vi "Configure View Model.vi"(8 "error in (no error)":errorcluster, 10 "View Model":refnum<class "Multicolumn List Box View Model.lvclass">, 11 "Multicolumn List Box View In":refnum<class "Multicolumn List Box View.lvclass">) -> (0 "error out":errorcluster, 3 "Multicolumn List Box View Out":refnum<class "Multicolumn List Box View.lvclass">)   [LabVIEW 2020, in "Multicolumn List Box View.lvclass"]
uses:
  Multicolumn List Box View.lvclass
  Multicolumn List Box View Model/Multicolumn List Box View Model.lvclass
  Multicolumn List Box View.lvclass/Multicolumn List Box View.ctl
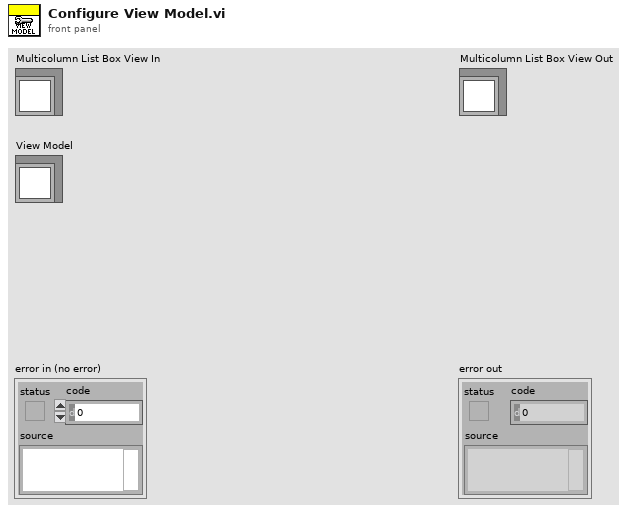
[diagram p1: front panel]
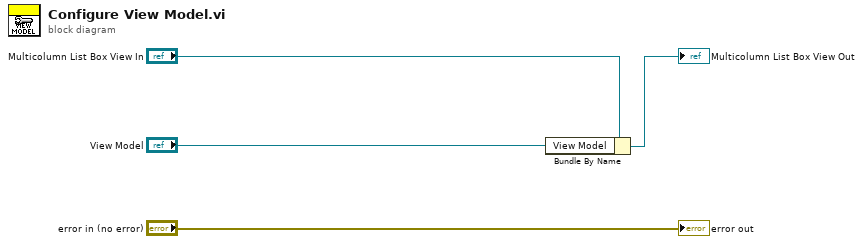
[diagram p0: block diagram]
diagram:
  n1 = Bundle By Name(cluster="Multicolumn List Box View In", "View Model"="View Model") -> (→"Multicolumn List Box View Out":refnum<class "Multicolumn List Box View.lvclass">)
  "error out" <- "error in (no error)"
